vi "GetPropertyValue.vi"(10 "Property":string, 11 "body":string) -> (3 "String out":string)   [LabVIEW 2021]
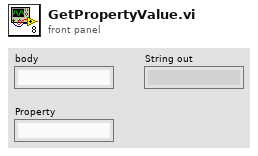
[diagram p1: front panel]
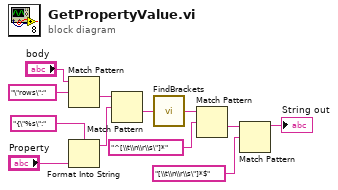
[diagram p0: block diagram]
diagram:
  n1 = Match Pattern(string="body", regular expression="\"rows\":") -> (after substring=w4:string)  [unwired: 1 in, 3 out]
  n2 = Format Into String(format string="{\"%s\":" ("regular expression"), "Property") -> (resulting string=w2:string)  [unwired: 2 in, 1 out]
  n3 = Match Pattern(string=w4, regular expression=w2) -> (after substring=w11:string)  [unwired: 1 in, 3 out]
  n4 = call "FindBrackets.vi"("String in"=w11) -> ("String out"=w12:string)
  n5 = Match Pattern(string=w12, regular expression="^[\\t\\n\\r\\s\"]*") -> (after substring=w8:string)  [unwired: 1 in, 3 out]
  n6 = Match Pattern(string=w8, regular expression="[\\t\\n\\r\\s\"]*$") -> (before substring=→"String out":string)  [unwired: 1 in, 3 out]
